vi "Create Test Configuration.vi"() -> (0 "error out":errorcluster, 1 "Names":string[](array[string]), 2 "Line Array":T1[](array[typedef]), 3 "Module Configuration":refnum<class "JSON_RPC_Interface configuration.lvclass">, 4 "Channels":refnum<class "TBM channel.lvclass">[](array[class]), 5 "instance identifier":string)   [LabVIEW 2017, in "JSON_RPC_Interface tests.lvlib"]
doc: "This VI creates a standard test configuration for other unit tests. It currently creates and adds one line with every datatype to the module configuration."
uses:
  JSON_RPC_Interface tests.lvlib
  module/configuration/JSON_RPC_Interface configuration.lvclass
  C:/Program Files (x86)/National Instruments/LabVIEW 2017/vi.lib/NI/Configuration Framework/serializable configuration/NISE_CEF_serializable configuration.lvclass
  module/configuration/Line.ctl
  <vilib>/NI/Tag Bus Module Framework/channel/TBM channel.lvclass
  <vilib>/NI/Tag Bus Module Framework/channel/channel classification.ctl
  <vilib>/NI/Configuration Framework/serializable configuration/NISE_CEF_serializable configuration.lvclass
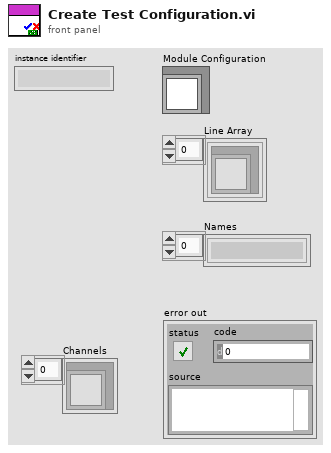
[diagram p1: front panel]
types:
  T1 = typedef "JSON_RPC_Interface configuration.lvclass/Line.ctl" = cluster{"channel":refnum<class "TBM channel.lvclass">}
  T2 = typedef "TBM channel.lvclass/channel classification.ctl" = enum16{"input data", "output data", "processing parameter", "processing result"}
  T3 = typedef "tag bus.lvlib/tag descriptor.lvclass/Data Type.ctl" = enum16{"Double", "Single", "I64", "I32", "I16", "I8", "U64", "U32", "U16", "U8", "Boolean", "String", "Array of Double", "Array of Single", "Array of I64", "Array of I32", "Array of I16", "Array of I8", "Array of U64", "Array of U32", "Array of U16", "Array of U8", "Array of Boolean", "Array of String"}
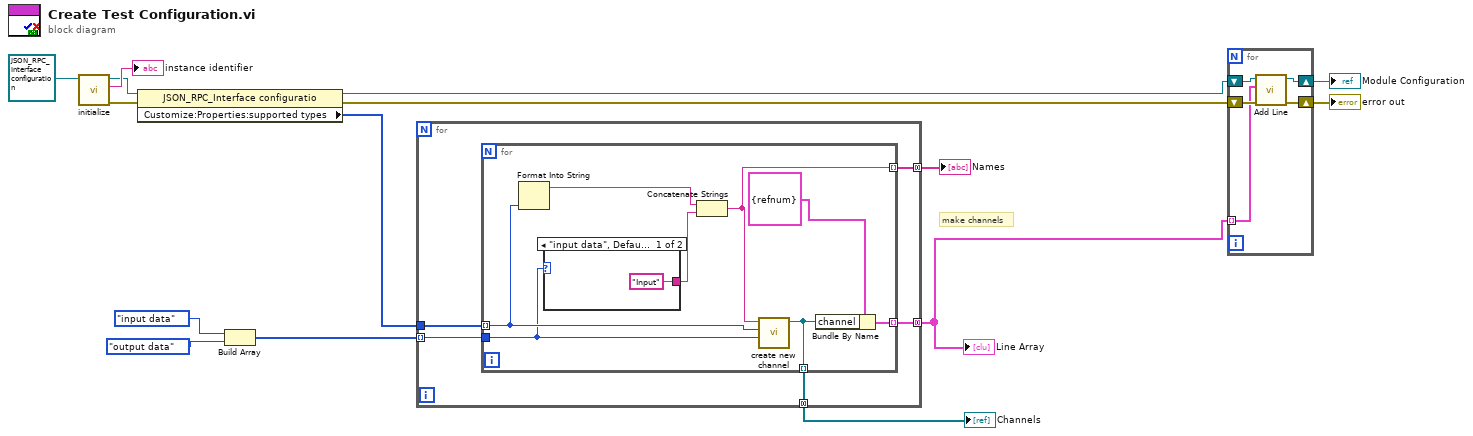
[diagram p0: block diagram]
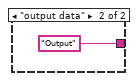
[diagram p2: hidden frame]
diagram:
  # "make channels"
  n1 = call <vilib>:"initialize.vi"("configuration in"=refnum<class "JSON_RPC_Interface configuration.lvclass"> refnum ("tag bus configurable plugin module configuration")) -> ("error out"=w13:errorcluster, "identifier"=→"instance identifier":string, "configuration out"=w10:refnum<class "JSON_RPC_Interface configuration.lvclass">)  [unwired: 8 in]
  n2 = property class="JSON_RPC_Interface configuratio"(reference=w10, error in=w13) -> (reference out=w6:refnum<class "JSON_RPC_Interface configuration.lvclass">, error out=w12:errorcluster, "Customize:Properties:supported types"=w7:T3[])
  n3 = Build Array(channel_classification."input data" ("channel classification"), channel_classification."output data" ("channel classification")) -> (w5:T2[])
  n4 = for {
    tunnel: w5 -> [w20] mode=indexing
    tunnel: [w18] -> w1 mode=concatenating
    tunnel: w7 -> [w19]
    tunnel: [w17] -> w11 mode=concatenating
    tunnel: [w16] -> w2 mode=concatenating
    n5 = for {
      tunnel: w20 -> [w24]
      tunnel: [w27] -> w18 mode=indexing
      tunnel: w19 -> [w25] mode=indexing
      tunnel: [w21] -> w17 mode=indexing
      tunnel: [w26] -> w16 mode=indexing
      n6 = Format Into String(w25) -> (resulting string=w23:string)  [unwired: 3 in, 1 out]
      n7 = case shown="\"input data\", Default" w24 {
        tunnel: ["Input" "Output"] -> w22
        frame "input data", Default {
        }
        frame "output data" {
        }
      }
      n8 = Concatenate Strings(w23, w22) -> (w21:string)
      n9 = call <vilib>:"create new channel.vi"("channel classification"=w24, "data type"=w25, "channel name"=w21) -> ("channel"=w26:refnum<class "TBM channel.lvclass">)  [unwired: 8 in]
      n10 = Bundle By Name(cluster=T1 {"channel"=refnum} ("Line"), "channel"=w26) -> (w27:T1)
    }
  }
  "Names" <- w11
  "Line Array" <- w1
  "Channels" <- w2
  n11 = for {
    tunnel: w1 -> [w31] mode=indexing
    shift-right: [w34] -> w9
    shift-left: w6 -> [w35]
    shift-right: [w32] -> w15
    shift-left: w12 -> [w33]
    n12 = call "Add Line.vi"("error in"=w33, "Line"=w31, "JSON_RPC_Interface configuration in"=w35) -> ("error out"=w32:errorcluster, "JSON_RPC_Interface configuration out"=w34:refnum<class "JSON_RPC_Interface configuration.lvclass">)  [unwired: 6 in, 1 out]
  }
  "error out" <- w15
  "Module Configuration" <- w9
